vi "PH_Periodic_Sequencer.Sequencer SM State.vi"(0 "i ref in":refnum<vi>, 2 "Service Name":string, 3 "SM State":string, 5 "error in (no error)":errorcluster) -> (14 "i ref out":refnum<vi>, 19 "error out":errorcluster)   [LabVIEW 2009]
doc: "This VI writes the state of the state machine of the related PU to own attributes and the GUI elements."
uses:
  PH_Sequencer/PH_Sequencer.lvlib
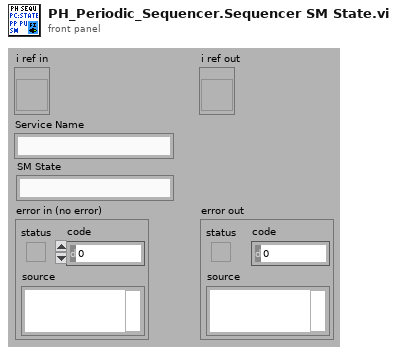
[diagram p1: front panel]
types:
  T1 = typedef "PH_Sequencer.lvlib/PH_Sequencer.i attribute.ctl" = cluster{"GUI Refs":cluster{"Main Off":refnum<vi>, "Fire":refnum<vi>, "Status":refnum<vi>, "Ready":refnum<vi>, "Waiting Time":refnum<vi>, "Timeout":refnum<vi>, "SMs ok":refnum<vi>, "PP DP Ready":refnum<vi>, "Sequencer SM State":refnum<vi>, "PP PA Ready":refnum<vi>, "Calorimeter":refnum<vi>, "Beamline Ready":refnum<vi>, "Clear Beamline":refnum<vi>, "Linkage PPMA Rods":refnum<vi>, "Linkage Current PA":refnum<vi>, "Linkage Current MA":refnum<vi>, "Linkage PPMA Rods 2":refnum<vi>, "Linkage PPMA Rods 3":refnum<vi>, "Linkage Current MA 2":refnum<vi>, "Linkage Current MA 3":refnum<vi>, "PP Booster Ready":refnum<vi>, "PP FR Ready":refnum<vi>, "Timing Ready":refnum<vi>, "State Timing":refnum<vi>, "Force Timing":refnum<vi>, "PSDB Shot Comment":refnum<vi>, "State PA Backreflection":refnum<vi>, "Beamline Z6 Ready":refnum<vi>, "Clear Z6 Beamline":refnum<vi>, "Sequence length":refnum<vi>, "Timing Mode":refnum<vi>, "Slow Trigger Settings":refnum<vi>, "Experiment Description":refnum<vi>, "State PSDB":refnum<vi>, "PSDB Ready":refnum<vi>, "Set PSDB Settings":refnum<vi>, "Get PSDB Info":refnum<vi>, "Take Snapshot":refnum<vi>, "Shottype":refnum<vi>, "Experiment":refnum<vi>, "PA Energy":refnum<vi>, "MA Energy":refnum<vi>, "MA Gain":refnum<vi>}, "Status Info":cluster{"Machine Status":T2, "WaitingTime":i32, "Timeout":bool}, "Readyness":cluster{"Ready to shot":bool, "PP DP Ready":bool, "PPPA Ready":bool, "BL Ready":bool, "PP Booster Ready":bool, "PP FR Ready":bool, "Timing Ready":bool, "BL Z6 Ready":bool, "PSDBReady":bool}, "Instancenames":cluster{"PPMA Rods":string, "PP Current Meas":string, "Beamline":string, "PA Backrefl Meas":string, "Beamline Z6":string}, "Data to read":bool, "Calorimeter":cluster{"Instancename":string, "On":bool, "linked":bool}, "Linkage":cluster{"PPMA Rods":bool, "PP Current Meas":bool, "Beamline":bool, "PA Backrefl Meas":bool, "Beamline Z6":bool}, "PU Info":T3[], "HV Info":T4[], "PSU Info":T5[], "Refs PU on":refnum<vi>[], "Refs Set Voltage PU":refnum<vi>[], "Refs State PU":refnum<vi>[], "Refs State SM PU":refnum<vi>[], "Refs Waiting Time PU":refnum<vi>[], "Refs TO SM PU":refnum<vi>[], "Refs Voltage PU":refnum<vi>[], "Timing":cluster{"Instance":string, "linked":bool, "Status":T2, "Timing Mode":T6, "Slow Trigger Settings":T7, "Info available":cluster{"ext SlowTrigger":bool, "T2":bool, "Mode":bool, "Delay Slow Trigger":bool}}, "GUI Manager Path":string, "Service ID R2S":i32, "PSDB":cluster{"Controller Instance":string, "Controller Status":T2, "Controller linked":bool, "Settings acknowledged":bool, "Current Experiment ID":i16, "Current Shot Type":i16, "Current Comment":string, "Remember Settings":bool, "Write 2 early":bool}, "PSDB Data":cluster{"Main Off?":bool, "Sequence Length":dbl, "Sequence startet":timestamp}, "Beamline":refnum<vi>[], "Powermeter":cluster{"PA":cluster{"Instance":string, "Energy [J]":dbl, "in use":bool}, "MA":cluster{"Instance":string, "Energy [J]":dbl, "in use":bool}, "MA Gain":dbl}}
  T2 = typedef "Status.ctl" = i16
  T3 = typedef "PH_Sequencer.lvlib/PH_Sequencer.PU Info.ctl" = cluster{"Instancename":string, "PU on":bool, "State":T2, "Waiting time":i32, "Set Voltage":dbl, "State SM":string, "Timeout SM":string, "linked":bool}
  T4 = typedef "PH_Sequencer.lvlib/PH_Sequencer.HV Meas Info.ctl" = cluster{"Instancename":string, "linked":bool, "Tagname Meas Voltage":string}
  T5 = typedef "PH_Sequencer.lvlib/PH_Sequencer.PSU Info.ctl" = cluster{"Instancename":string, "linked":bool, "Tagname Applied Voltage":string}
  T6 = typedef "PH_Timing.lvlib/PH_Timing.Timing Mode.ctl" = cluster{"T2 [s]":i16, "Modeselector":enum32{"10 Hz", "0.5 Hz", "Shot"}}
  T7 = typedef "PH_Timing.lvlib/PH_Timing.Slow Trigger Settings.ctl" = cluster{"Delay [ms]":dbl, "externally triggered?":bool}
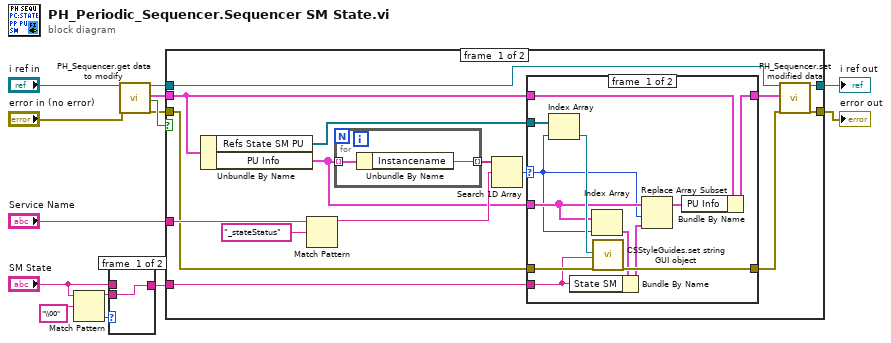
[diagram p0: block diagram]
diagram:
  n1 = Match Pattern(string="SM State", regular expression="\\00" ("search string")) -> (before substring=w1:string, offset past match=w4:i32)  [unwired: 1 in, 2 out]
  n2 = case shown="-1" w4 {
    tunnel: [w15 w16] -> w2
    tunnel: "SM State" -> [_ w16]
    tunnel: w1 -> [w15 _]
    frame #0 {
    }
    frame #1 {
    }
  }
  n3 = call "PH_Sequencer.get data to modify.vi"("i ref in"="i ref in", "error in (no error)"="error in (no error)") -> ("i ref out"=w8:refnum<vi>, "i attribute"=w12:T1, "timed out"=w14:bool, "error out"=w10:errorcluster)  [unwired: 14 in]
  n4 = case shown="False" w14 {
    tunnel: w8 -> [w17 w49]
    tunnel: [w31 w49] -> w9
    tunnel: w10 -> [w23 w48]
    tunnel: [w30 w48] -> w11
    tunnel: w12 -> [w18 _]
    tunnel: w2 -> [w20 _]
    tunnel: "Service Name" -> [w28 _]
    frame #0 {
      n5 = Unbundle By Name(w18) -> ("Refs State SM PU"=w21:refnum<vi>[], "PU Info"=w19:T3[])
      n6 = Match Pattern(string=w28, regular expression="_stateStatus") -> (before substring=w26:string)  [unwired: 1 in, 3 out]
      n7 = for {
        tunnel: w19 -> [w47] mode=indexing
        tunnel: [w46] -> w27 mode=indexing
        n8 = Unbundle By Name(w47) -> ("Instancename"=w46:string)
      }
      n9 = Search 1D Array(1D array=w27, element=w26) -> (index of element=w25:i32)  [unwired: 1 in]
      n10 = case shown="Default" w25 {
        selector: w25 -> [w35 _]
        tunnel: [w32 w44] -> w24
        tunnel: [w40 w45] -> w22
        tunnel: w23 -> [w41 w45]
        tunnel: w21 -> [w43 _]
        tunnel: w20 -> [w38 _]
        tunnel: w19 -> [w37 _]
        tunnel: w18 -> [w33 w44]
        frame #0 {
          n11 = Index Array(array=w43, index=w35) -> (element=w42:refnum<vi>)
          n12 = Index Array(array=w37, index=w35) -> (element=w39:T3)
          n13 = Bundle By Name(cluster=w39, "State SM"=w38) -> (w36:T3)
          n14 = call "CSStyleGuides.set string GUI object.vi"("GUI object Ref"=w42, "Text"=w38, "error in (no error)"=w41) -> ("error out"=w40:errorcluster)  [unwired: 16 in]
          n15 = Replace Array Subset(array=w37, new element=w36, index=w35) -> (w34:T3[])
          n16 = Bundle By Name(cluster=w33, "PU Info"=w34) -> (w32:T1)
        }
        frame #1 {
        }
      }
      n17 = call "PH_Sequencer.set modified data.vi"("i ref in"=w17, "i attribute"=w24, "error in (no error)"=w22) -> ("i ref out"=w31:refnum<vi>, "error out"=w30:errorcluster)  [unwired: 15 in]
    }
    frame #1 {
    }
  }
  "error out" <- w11
  "i ref out" <- w9
